vi "add_time_roslv.vi"   [LabVIEW 2014]
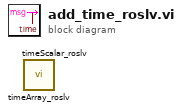
[diagram p0: block diagram]
diagram:
  n1 = call "timeArray_roslv.vi"() -> ()  [unwired: 5 in, 1 out]
  n2 = call "timeScalar_roslv.vi"() -> ()  [unwired: 5 in, 1 out]
